vi "testi4.vi"() -> ()   [LabVIEW 2015]
uses:
  BERTTA.dll
panel:
  out "rc":i32
  out "save data":dbl
  out "Lauda":dbl
  in  "Set Lauda":dbl
  out "Mettler 2":dbl
  out "Mettler 1":dbl
  in  "Set Heidolph":i32
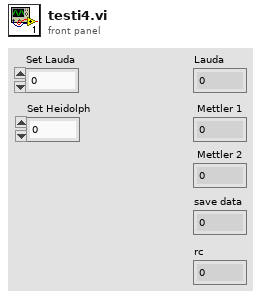
[diagram p1: front panel]
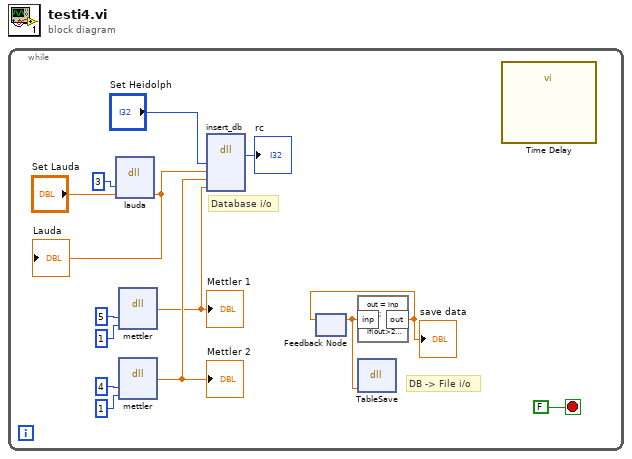
[diagram p0: block diagram]
diagram:
  n1 = while {
    stop <- FALSE stop-if-true
    # "DB -> File i/o"
    # "Database i/o"
    n2 = dll-call lib="C:/Users/xlaraser/Documents/Visual Studio 2017/Projects/Bertta/BERTTA/Debug/BERTTA.dll" fn="lauda"("port"=3, "set_temp"="Set Lauda") -> ("set_temp"=w6:dbl)  [unwired: 5 in, 2 out]
    "Lauda" <- w6
    n3 = dll-call lib="C:/Users/xlaraser/Documents/Visual Studio 2017/Projects/Bertta/BERTTA/Debug/BERTTA.dll" fn="mettler"("port"=5, "msg"=1) -> ("return type"=w11:dbl)  [unwired: 5 in, 2 out]
    "Mettler 1" <- w11
    n4 = dll-call lib="C:/Users/xlaraser/Documents/Visual Studio 2017/Projects/Bertta/BERTTA/Debug/BERTTA.dll" fn="mettler"("port"=4, "msg"=1) -> ("return type"=w12:dbl)  [unwired: 5 in, 2 out]
    "Mettler 2" <- w12
    n5 = dll-call lib="C:/Users/xlaraser/Documents/Visual Studio 2017/Projects/Bertta/BERTTA/Debug/BERTTA.dll" fn="insert_db"("heidolph"="Set Heidolph", "lauda"=w6, "mettler1"=w12, "mettler2"=w11) -> ("return type"=→"rc":i32)  [unwired: 7 in, 2 out]
    n6 = feedback #1() -> (w2:dbl)  [unwired: 1 in]
    n7 = formula code="out = inp + 1;\n\nif(out>20) out = 0;"("inp"=w2) -> ("out"=w3:dbl)
    "save data" <- w3
    n8 = feedback-in #1(w3) -> ()
    n9 = dll-call lib="C:/Users/xlaraser/Documents/Visual Studio 2017/Projects/Bertta/BERTTA/Debug/BERTTA.dll" fn="TableSave"("exec"=w2) -> ()  [unwired: 5 in, 2 out]
    n10 = call "Time Delay"() -> ()  [unwired: 11 in, 1 out]
  }
